vi "OP600ZP_INTLCK_LOOP.vi"(8 "entrée d'erreur (pas d'erreur)":errorcluster) -> (0 "sortie d'erreur":errorcluster, 1 "Chaîne 2":string, 2 "Chaîne 3":string, 3 "Case à cocher":bool, 4 "Chaîne":string, 5 "cas vrai":string)   [LabVIEW 2020]
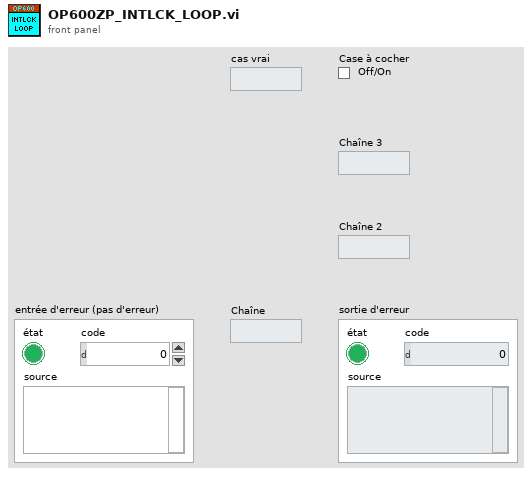
[diagram p1: front panel]
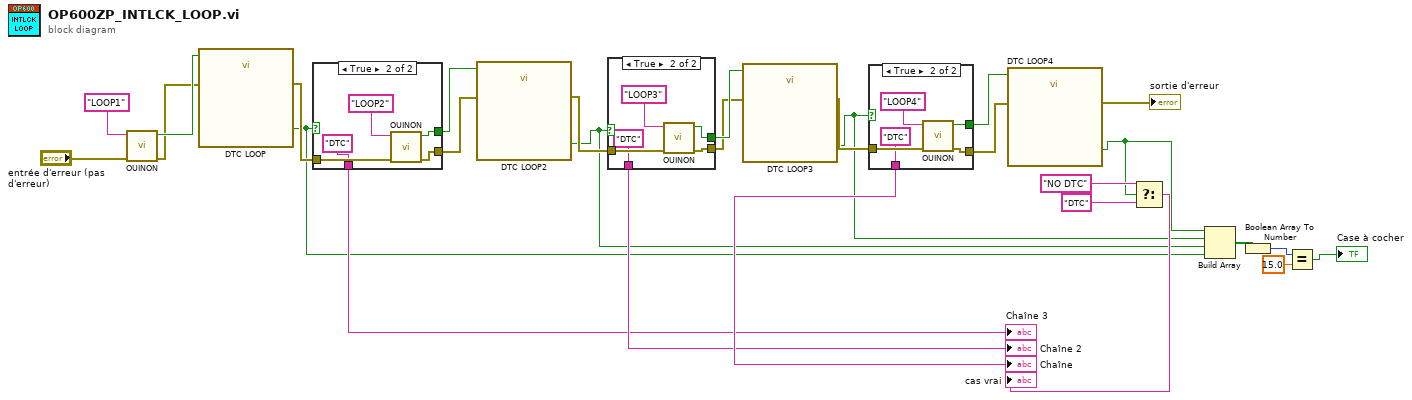
[diagram p0: block diagram]
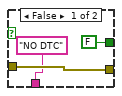
[diagram p2: hidden frame]
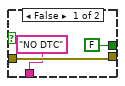
[diagram p3: hidden frame]
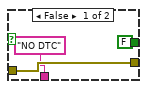
[diagram p4: hidden frame]
diagram:
  n1 = call "OUINON.vi"("errin"="entrée d'erreur (pas d'erreur)", "image"="LOOP1" ("IN")) -> ("error out"=w7:errorcluster, "OUI/NON"=w21:bool)  [unwired: 8 in]
  n2 = call "DTC LOOP"("Enable"=w21, "error in (no error)"=w7) -> ("Y'a t-il des DTC?"=w1:bool, "error out"=w8:errorcluster)  [unwired: 15 in, 1 out]
  n3 = case shown="True" w1 {
    tunnel: w8 -> [w31 w35]
    tunnel: [FALSE ("OUI/NON") w34] -> w24
    tunnel: [w31 w33] -> w9
    tunnel: ["NO DTC" "DTC"] -> w15
    frame False {
    }
    frame True {
      n4 = call "OUINON.vi"("errin"=w35, "image"="LOOP2" ("IN")) -> ("error out"=w33:errorcluster, "OUI/NON"=w34:bool)  [unwired: 8 in]
    }
  }
  "Chaîne 3" <- w15
  n5 = call "DTC LOOP2"("Enable"=w24, "error in (no error)"=w9) -> ("Y'a t-il des DTC?"=w2:bool, "error out"=w10:errorcluster)  [unwired: 15 in, 1 out]
  n6 = case shown="True" w2 {
    tunnel: w10 -> [w38 w43]
    tunnel: [w38 w42] -> w11
    tunnel: [FALSE ("OUI/NON") w41] -> w23
    tunnel: ["NO DTC" "DTC"] -> w16
    frame False {
    }
    frame True {
      n7 = call "OUINON.vi"("errin"=w43, "image"="LOOP3" ("IN")) -> ("error out"=w42:errorcluster, "OUI/NON"=w41:bool)  [unwired: 8 in]
    }
  }
  "Chaîne 2" <- w16
  n8 = call "DTC LOOP3"("Enable"=w23, "error in (no error)"=w11) -> ("Y'a t-il des DTC?"=w3:bool, "error out"=w12:errorcluster)  [unwired: 15 in, 1 out]
  n9 = case shown="True" w3 {
    tunnel: w12 -> [w47 w51]
    tunnel: [w47 w50] -> w13
    tunnel: [FALSE ("OUI/NON") w49] -> w22
    tunnel: ["NO DTC" "DTC"] -> w17
    frame False {
    }
    frame True {
      n10 = call "OUINON.vi"("errin"=w51, "image"="LOOP4" ("IN")) -> ("error out"=w50:errorcluster, "OUI/NON"=w49:bool)  [unwired: 8 in]
    }
  }
  "Chaîne" <- w17
  n11 = call "DTC LOOP4"("Enable"=w22, "error in (no error)"=w13) -> ("Absence de DTC?"=w4:bool, "error out"=→"sortie d'erreur":errorcluster)  [unwired: 15 in, 1 out]
  n12 = Select(t="NO DTC" ("cas vrai"), s=w4, f="DTC") -> (s? t:f=→"cas vrai":string)
  n13 = Build Array(w4, w3, w2, w1) -> (w25:bool[])
  n14 = Boolean Array To Number(Boolean array=w25) -> (number=w27:u32)
  n15 = Equal?(x=w27, y=15.0) -> (x = y?=→"Case à cocher":bool)
